vi "NIIE_ListGlyphsAndTemplates.vi"(8 "Error":errorcluster, 11 "Data":T1={"Class"={"Ants"=refnum, "Layer"=refnum, "Templates"=refnum, "Icon"=refnum, "Glyph"=refnum, "Settings"=refnum, "Tools"=refnum}, "Ref"={"Add Layer"=refnum, "Remove Layer"=refnum, "Line Text"=[], "Body Text Spec"=refnum, "DNL_Font"=refnum, "glyph path str"=refnum, "templates path str"=refnum, "Arrow Up"=refnum, "Arrow Down"=refnum, "IE VI Ref"=refnum, "Glyphs tree"=refnum, "Templates tree"=refnum, "Layer Icon Text"=refnum, "Layer Template"=refnum, "Clipboard"=refnum, "BW icon in"=refnum, "Color icon in"=refnum, "Layer Clust"=refnum, "Body Text"=refnum, "DNL_Framework Templates"=refnum, "Search Templates"=refnum, "TextMarker"=refnum, "Tab Control"=refnum, "Search Glyphs"=refnum, "Line Color"=refnum, "DNL_Glyphs []"=refnum, "Fill Color"=refnum, "Tools"=refnum, "Glyphs tree"=refnum, "Icon"=refnum, "Preview"=refnum, "Ants"=refnum, "Terminals"=refnum, "menu reference"=refnum, "LayerNames"=[], "GlyphLoadAnimation"=refnum, "TemplateLoadAnimation"=refnum, "refreshGlyphs"=refnum, "refreshTemplates"=refnum}, "Support"={"AntsRect"={"left"=0, "top"=0, "right"=0, "bottom"=0}, "Mouse Move Coords"={"Horizontal"=0, "Vertical"=0}, "Mouse Down Coords"={"Horizontal"=0, "Vertical"=0}, "Temp Coord"={"Horizontal"=0, "Vertical"=0}, "Action"=enum."Default", "Edge Color"=4914962, "Fill Color"=16860, "Mouse Down?"=FALSE, "Draft Mode?"=FALSE, "Temp Icon"=bytes[3102], "CTRL Pressed"=FALSE, "Move Selection?"=FALSE, "AntsRect Orig"={"left"=0, "top"=0, "right"=0, "bottom"=0}, "Text"="", "TM Set?"=FALSE, "Mouse inside icon?"=FALSE, "Tool (old value)"=0, "Pencil Move Color"=0, "Swap Colors?"=FALSE, "Shift pressed?"=FALSE}}) -> (0 "Error Out":errorcluster={"status"=TRUE, "code"=7, "source"="Open/Create/Replace File in Read Glyphs from  File.vi->ListGlyphsAndTemplates.vi<APPEND>\nC:\\Documents and Settings\\grsandrt\\My Documents\\LabVIEW Data\\Icon Templates\\Library\\Templates.8.6f1.bin"}, 3 "Data Out":T1={"Class"={"Ants"=refnum, "Layer"=refnum, "Templates"=refnum, "Icon"=refnum, "Glyph"=refnum, "Settings"=refnum, "Tools"=refnum}, "Ref"={"Add Layer"=refnum, "Remove Layer"=refnum, "Line Text"=[], "Body Text Spec"=refnum, "DNL_Font"=refnum, "glyph path str"=refnum, "templates path str"=refnum, "Arrow Up"=refnum, "Arrow Down"=refnum, "IE VI Ref"=refnum, "Glyphs tree"=refnum, "Templates tree"=refnum, "Layer Icon Text"=refnum, "Layer Template"=refnum, "Clipboard"=refnum, "BW icon in"=refnum, "Color icon in"=refnum, "Layer Clust"=refnum, "Body Text"=refnum, "DNL_Framework Templates"=refnum, "Search Templates"=refnum, "TextMarker"=refnum, "Tab Control"=refnum, "Search Glyphs"=refnum, "Line Color"=refnum, "DNL_Glyphs []"=refnum, "Fill Color"=refnum, "Tools"=refnum, "Glyphs tree"=refnum, "Icon"=refnum, "Preview"=refnum, "Ants"=refnum, "Terminals"=refnum, "menu reference"=refnum, "LayerNames"=[], "GlyphLoadAnimation"=refnum, "TemplateLoadAnimation"=refnum, "refreshGlyphs"=refnum, "refreshTemplates"=refnum}, "Support"={"AntsRect"={"left"=0, "top"=0, "right"=0, "bottom"=0}, "Mouse Move Coords"={"Horizontal"=0, "Vertical"=0}, "Mouse Down Coords"={"Horizontal"=0, "Vertical"=0}, "Temp Coord"={"Horizontal"=0, "Vertical"=0}, "Action"=enum."Default", "Edge Color"=4914962, "Fill Color"=16860, "Mouse Down?"=FALSE, "Draft Mode?"=FALSE, "Temp Icon"=bytes[3102], "CTRL Pressed"=FALSE, "Move Selection?"=FALSE, "AntsRect Orig"={"left"=0, "top"=0, "right"=0, "bottom"=0}, "Text"="", "TM Set?"=FALSE, "Mouse inside icon?"=FALSE, "Tool (old value)"=0, "Pencil Move Color"=0, "Swap Colors?"=FALSE, "Shift pressed?"=FALSE}})   [LabVIEW 2021]
uses:
  Controls/IE Data.ctl
  Class/Ants/Ants.lvclass
  Class/FakedArray/FakedArray.lvclass
  Class/Icon Library/Glyph.lvclass
  Class/Settings/Settings.lvclass
  Class/Tools/Tools Paint.lvclass
  vi.lib/LabVIEW Icon API/lv_icon/Classes/Icon/Icon.lvclass
  Controls/IE Classes.ctl
  Controls/References Cluster.ctl
  Controls/SupportClass.ctl
  <vilib>/Utility/miscctls.llb/LVPoint32TypeDef.ctl
  Controls/ENUM_SupportClass_Action.ctl
  vi.lib/LabVIEW Icon API/lv_icon/Controls/IEColor.ctl
  vi.lib/LabVIEW Icon API/lv_icon/Controls/Pathes.ctl
  vi.lib/LabVIEW Icon API/lv_icon/lv_icon.lvlib
panel:
  in  "Template Header":string="Icon Templates"
  in  "Glyphs Header":string="Glyphs"
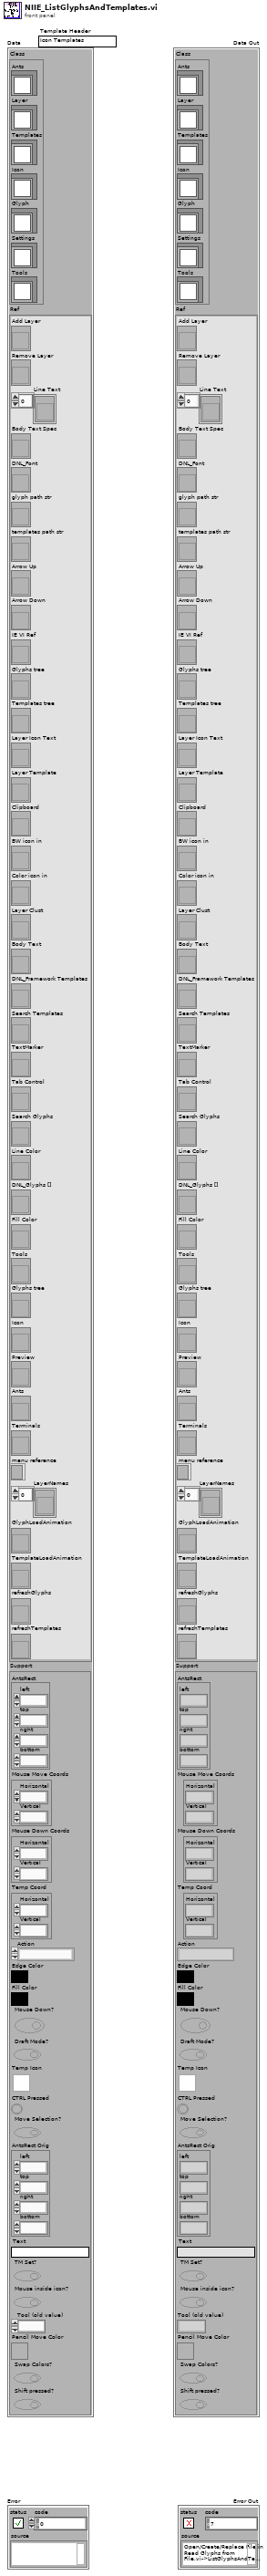
[diagram p1: front panel]
types:
  T1 = typedef "IE Data.ctl" = cluster{"Class":T2, "Ref":T3, "Support":T4}
  T2 = typedef "IE Classes.ctl" = cluster{"Ants":refnum<class "Ants.lvclass">, "Layer":refnum<class "FakedArray.lvclass">, "Templates":refnum<class "FakedArray.lvclass">, "Icon":refnum<class "Icon.lvclass">, "Glyph":refnum<class "Glyph.lvclass">, "Settings":refnum<class "Settings.lvclass">, "Tools":refnum<class "Tools Paint.lvclass">}
  T3 = typedef "References Cluster.ctl" = cluster{"Add Layer":refnum<vi>, "Remove Layer":refnum<vi>, "Line Text":refnum<vi>[], "Body Text Spec":refnum<vi>, "DNL_Font":refnum<vi>, "glyph path str":refnum<vi>, "templates path str":refnum<vi>, "Arrow Up":refnum<vi>, "Arrow Down":refnum<vi>, "IE VI Ref":refnum<vi>, "Glyphs tree":refnum<vi>, "Templates tree":refnum<vi>, "Layer Icon Text":refnum<vi>, "Layer Template":refnum<vi>, "Clipboard":refnum<vi>, "BW icon in":refnum<vi>, "Color icon in":refnum<vi>, "Layer Clust":refnum<vi>, "Body Text":refnum<vi>, "DNL_Framework Templates":refnum<vi>, "Search Templates":refnum<vi>, "TextMarker":refnum<vi>, "Tab Control":refnum<vi>, "Search Glyphs":refnum<vi>, "Line Color":refnum<vi>, "DNL_Glyphs []":refnum<vi>, "Fill Color":refnum<vi>, "Tools":refnum<vi>, "Glyphs tree":refnum<vi>, "Icon":refnum<vi>, "Preview":refnum<vi>, "Ants":refnum<vi>, "Terminals":refnum<vi>, "menu reference":refnum<k9>, "LayerNames":refnum<vi>[], "GlyphLoadAnimation":refnum<vi>, "TemplateLoadAnimation":refnum<vi>, "refreshGlyphs":refnum<vi>, "refreshTemplates":refnum<vi>}
  T4 = typedef "SupportClass.ctl" = cluster{"AntsRect":cluster{"left":i16, "top":i16, "right":i16, "bottom":i16}, "Mouse Move Coords":T5, "Mouse Down Coords":T5, "Temp Coord":T5, "Action":T6, "Edge Color":T7, "Fill Color":T7, "Mouse Down?":bool, "Draft Mode?":bool, "Temp Icon":picture, "CTRL Pressed":bool, "Move Selection?":bool, "AntsRect Orig":cluster{"left":i16, "top":i16, "right":i16, "bottom":i16}, "Text":string, "TM Set?":bool, "Mouse inside icon?":bool, "Tool (old value)":u32, "Pencil Move Color":u32, "Swap Colors?":bool, "Shift pressed?":bool}
  T5 = typedef "LVPoint32TypeDef.ctl" = cluster{"Horizontal":i32, "Vertical":i32}
  T6 = typedef "ENUM_SupportClass_Action.ctl" = enum16{"Default", "Move Selection", "Glyph Library", "Tool"}
  T7 = typedef "IEColor.ctl" = u32
  T8 = typedef "Pathes.ctl" = enum16{"Root Path", "Icon Templates", "Icon Templates VI", "Icon Templates Lib", "Glyphs"}
  T9 = typedef "Cluster_Path&Icon.ctl" = cluster{"Rectangle":cluster{"left":i16, "top":i16, "right":i16, "bottom":i16}, "Path":path, "Image":picture, "Filter":string, "FileName":string}
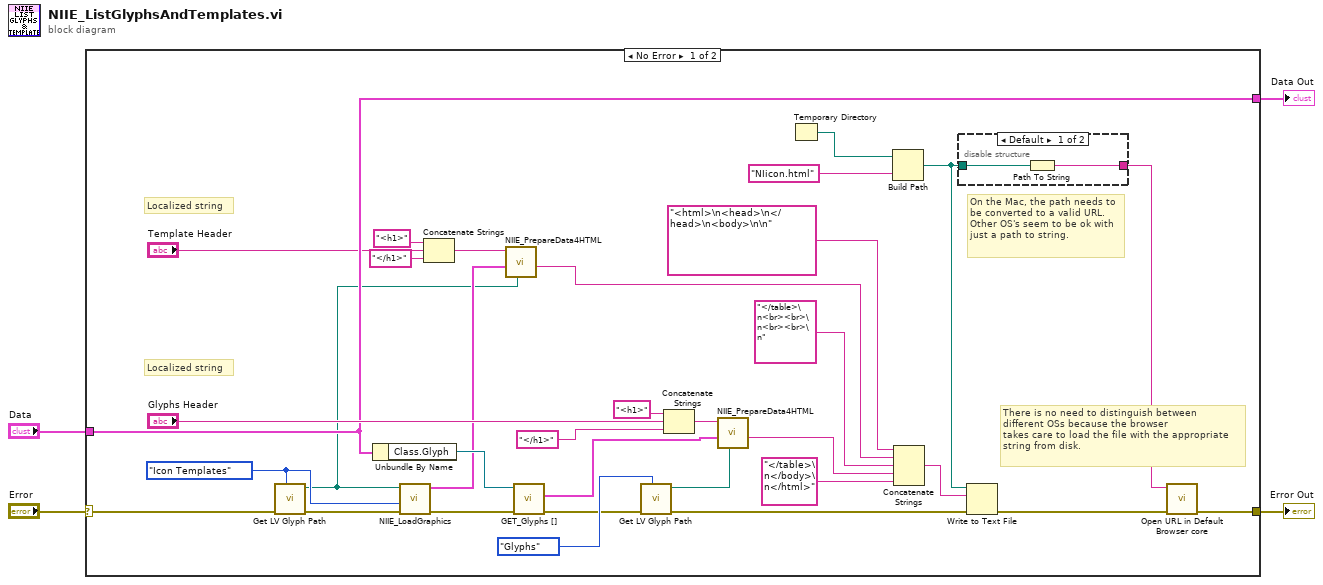
[diagram p0: block diagram]
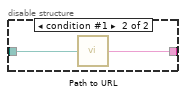
[diagram p2: hidden frame]
diagram:
  n1 = case shown="No Error" "Error" {
    selector: "Error" -> [w5 w43]
    tunnel: [w25 w43] -> w3
    tunnel: "Data" -> [w22 w42]
    tunnel: [w22 w42] -> w1
    frame No Error {
      w14 = Pathes."Icon Templates" ("Path")
      # "On the Mac, the path needs to be converted to a valid URL. Other OS's seem to be ok with just a path to string."
      # "There is no need to distinguish between\ndifferent OSs because the browser\ntakes care to load the file with the appropriate\nstring from disk."
      # "Localized string"
      # "Localized string"
      n2 = call "Get LV Glyph Path.vi"("Path"=w14, "error in (no error)"=w5) -> ("error out"=w15:errorcluster, "Requested Path"=w12:path)  [unwired: 1 in, 7 out]
      n3 = Unbundle By Name(w22) -> ("Class.Glyph"=w23:refnum<class "Glyph.lvclass">)
      n4 = call "NIIE_LoadGraphics.vi"("Error"=w15, "Source"=w14, "Graphic Root Folder"=w12) -> ("Error Out"=w8:errorcluster, "Glyphs Out"=w13:T9[])  [unwired: 3 in, 4 out]
      n5 = Concatenate Strings("<h1>" ("Header"), "Template Header", "</h1>" ("Header")) -> (w18:string)
      n6 = call "NIIE_PrepareData4HTML.vi"("Root"=w12, "Glyphs []"=w13, "Header"=w18) -> ("HTML String Out"=w10:string)  [unwired: 8 out]
      n7 = call-dynamic "GET_Glyphs [].vi"("Error"=w8, "Glyph.lvclass"=w23) -> ("Error Out"=w7:errorcluster, "Glyphs [] Out"=w32:T9[])  [unwired: 8 out]
      n8 = call "Get LV Glyph Path.vi"("Path"=Pathes."Glyphs", "error in (no error)"=w7) -> ("error out"=w6:errorcluster, "Requested Path"=w17:path)  [unwired: 1 in, 7 out]
      n9 = Concatenate Strings("<h1>" ("Header"), "Glyphs Header", "</h1>" ("Header")) -> (w27:string)
      n10 = call "NIIE_PrepareData4HTML.vi"("Root"=w17, "Glyphs []"=w32, "Header"=w27) -> ("HTML String Out"=w31:string)  [unwired: 8 out]
      n11 = Temporary Directory() -> (w34:path)
      n12 = Build Path(base path=w34, name or relative path="NIicon.html") -> (appended path=w36:path)
      n13 = Concatenate Strings("<html>\n<head>\n</head>\n<body>\n\n", w10, "</table>\n<br><br>\n<br><br>\n", w31, "</table>\n</body>\n</html>") -> (w33:string)
      n14 = disable-structure shown="Default" {
        disable-tunnel: w36 -> [w39 w41]
        disable-tunnel: [w38 w40] -> w24
        frame condition #0 (active) {
          n15 = Path To String(path=w39) -> (string=w38:string)
        }
        frame condition #1 {
          n16 = call <vilib>:"Path to URL.vi"("path"=w41) -> ("url"=w40:string)
        }
      }
      n17 = Write to Text File(file (use dialog)=w36, text=w33, error in=w6) -> (error out=w26:errorcluster)  [unwired: 3 out]
      n18 = call <vilib>:"Open URL in Default Browser core.vi"("error in (no error)"=w26, "url"=w24) -> ("error out"=w25:errorcluster)  [unwired: 5 out]
    }
    frame Error {
    }
  }
  "Error Out" <- w3
  "Data Out" <- w1
